vi "roboRIO v1.0 Shutdown Relay.vi"(8 "error in (no error)":errorcluster, 10 "Channel List":T3, 11 "myRIO Ref In":T1) -> (0 "error out":errorcluster, 3 "myRIO Ref Out":T1)   [LabVIEW 2021]
uses:
  <vilib>/myRIO/Common/Instrument Driver Framework/roboRIO v1.0/Relay/typedefs/Relay Channels List.ctl
  <vilib>/myRIO/Common/Instrument Driver Framework/roboRIO v1.0/Relay/typedefs/Relay Channels Enum.ctl
  <vilib>/myRIO/Common/Instrument Driver Framework/Utilities/typedefs/myRIO v1.0 Reference.ctl
  <vilib>/myRIO/Common/Instrument Driver Framework/Utilities/typedefs/Generic FPGA Reference.ctl
  <vilib>/myRIO/Common/Instrument Driver Framework/roboRIO v1.0/Relay/typedefs/Relay FPGA Reference.ctl
  <vilib>/Utility/error.llb/Error Cluster From Error Code.vi
  <vilib>/rvi/errors/niLvFpgaAdjustHostInterfaceError.vi
  <vilib>/rvi/interface/nirviReadWriteControl/nirviReadWriteControl.xnode
  NiFpgaLv.dll
  <vilib>/rvi/interface/Simulation/niFpgaSimulationCallBeginRW.vi
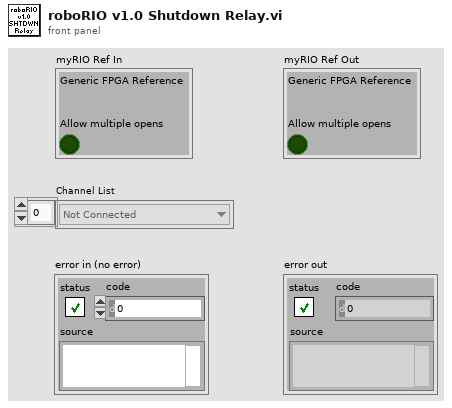
[diagram p1: front panel]
types:
  T1 = typedef "myRIO v1.0 Reference.ctl" = cluster{"Generic FPGA Reference":T2, "Allow multiple opens":bool}
  T2 = typedef "Generic FPGA Reference.ctl" = refnum<k20>
  T3 = typedef "Relay Channels List.ctl" = T4[]
  T4 = typedef "Relay Channels Enum.ctl" = enum16{"Not Connected", "RELAY/RELAY0", "RELAY/RELAY1", "RELAY/RELAY2", "RELAY/RELAY3"}
  T5 = typedef "Relay FPGA Reference.ctl" = refnum<k20>
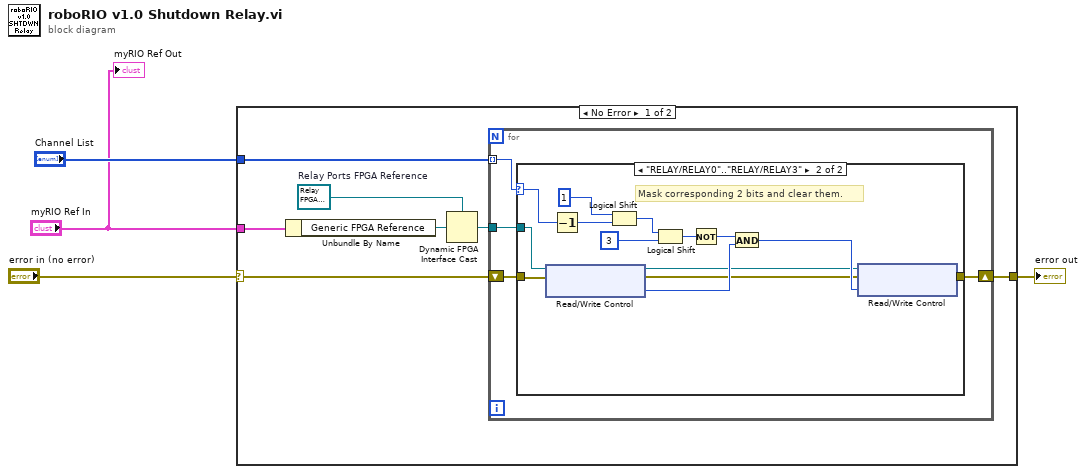
[diagram p0: block diagram]
diagram:
  n1 = case shown="No Error" "error in (no error)" {
    selector: "error in (no error)" -> [w8 w31]
    tunnel: "myRIO Ref In" -> [w7 _]
    tunnel: [w9 w31] -> w3
    tunnel: "Channel List" -> [w5 _]
    frame No Error {
      w11 = T5 refnum  # Relay Ports FPGA Reference
      n2 = Unbundle By Name(w7) -> ("Generic FPGA Reference"=w6:T2)
      n3 = Dynamic FPGA Interface Cast(Session In=w11, Type=w6) -> (Session Out=w10:T5)
      n4 = for {
        tunnel: w5 -> [w12] mode=indexing
        tunnel: w10 -> [w15]
        shift-right: [w14] -> w9
        shift-left: w8 -> [w13]
        n5 = case shown="\"RELAY/RELAY0\"..\"RELAY/RELAY3\"" w12 {
          selector: w12 -> [_ w17]
          tunnel: w15 -> [_ w29]
          tunnel: [w16 w30] -> w14
          tunnel: w13 -> [w16 w28]
          frame "Not Connected", Default {
          }
          frame "RELAY/RELAY0".."RELAY/RELAY3" {
            # "Mask corresponding 2 bits and clear them."
            n6 = xnode "Read/Write Control"("FPGA VI Reference In"=w29, "error in"=w28) -> ("FPGA VI Reference Out"=w19:T5, "error out"=w20:errorcluster, "DO.RELAY.OUT"=w22:u8)
            n7 = Decrement(x=w17) -> (x-1=w18:T4)
            n8 = Logical Shift(y=i16 1, x=w18) -> (x << y=w26:u32)
            n9 = Logical Shift(y=w26, x=u8 3) -> (x << y=w24:u8)
            n10 = Not(x=w24) -> (.not. x?=w23:u8)
            n11 = And(x=w23, y=w22) -> (x .and. y?=w21:u8)
            n12 = xnode "Read/Write Control"("FPGA VI Reference In"=w19, "error in"=w20, "DO.RELAY.OUT"=w21) -> ("error out"=w30:errorcluster)  [unwired: 1 out]
          }
        }
      }
    }
    frame Error {
    }
  }
  "error out" <- w3
  "myRIO Ref Out" <- "myRIO Ref In"
